vi "VI-Create XControl Event Generation.vi"(0 "Path":path=path "C:/Users/hancock/Desktop/Test/Test.xctl", 11 "error in (no error)":errorcluster) -> (15 "error out":errorcluster)   [LabVIEW 2015]
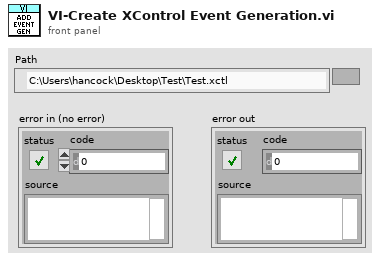
[diagram p1: front panel]
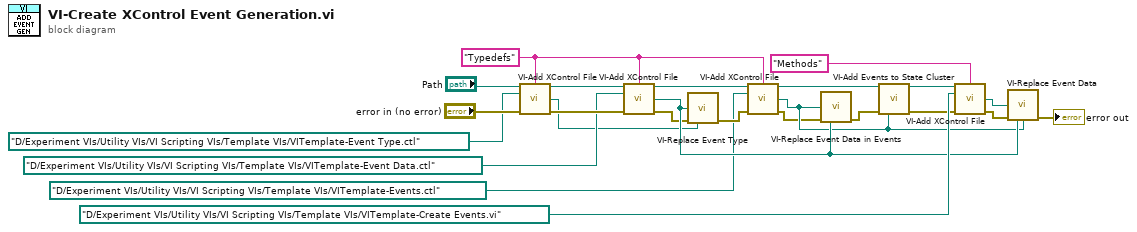
[diagram p0: block diagram]
diagram:
  w4 = "Typedefs"
  n1 = call "VI-Add XControl File.vi"("XCtl Path in"="Path", "Add to folder"=w4, "Template"=path "D:/Experiment VIs/Utility VIs/VI Scripting VIs/Template VIs/VITemplate-Event Type.ctl", "error in (no error)"="error in (no error)") -> ("XCtl Path out"=w12:path, "local path"=w8:path, "error out"=w11:errorcluster)  [unwired: 9 in]
  n2 = call "VI-Add XControl File.vi"("XCtl Path in"=w12, "Add to folder"=w4, "Template"=path "D:/Experiment VIs/Utility VIs/VI Scripting VIs/Template VIs/VITemplate-Event Data.ctl", "error in (no error)"=w11) -> ("XCtl Path out"=w7:path, "local path"=w17:path, "error out"=w9:errorcluster)  [unwired: 9 in]
  n3 = call "VI-Replace Event Type.vi"("Event Data typedef"=w17, "error in (no error)"=w9, "Event Type typedef"=w8) -> ("error out"=w6:errorcluster)  [unwired: 12 in]
  n4 = call "VI-Add XControl File.vi"("XCtl Path in"=w7, "Add to folder"=w4, "Template"=path "D:/Experiment VIs/Utility VIs/VI Scripting VIs/Template VIs/VITemplate-Events.ctl", "error in (no error)"=w6) -> ("XCtl Path out"=w1:path, "local path"=w16:path, "error out"=w3:errorcluster)  [unwired: 9 in]
  n5 = call "VI-Replace Event Data in Events.vi"("Events typedef"=w16, "error in (no error)"=w3, "Event Data typedef"=w17) -> ("error out"=w2:errorcluster)  [unwired: 12 in]
  n6 = call "VI-Add Events to State Cluster.vi"("XCtl Path in"=w1, "error in (no error)"=w2, "Event Data typedef"=w16) -> ("XCtl Path out"=w19:path, "error out"=w18:errorcluster)  [unwired: 11 in]
  n7 = call "VI-Add XControl File.vi"("XCtl Path in"=w19, "Add to folder"="Methods", "Template"=path "D:/Experiment VIs/Utility VIs/VI Scripting VIs/Template VIs/VITemplate-Create Events.vi", "error in (no error)"=w18) -> ("local path"=w22:path, "error out"=w21:errorcluster)  [unwired: 9 in, 1 out]
  n8 = call "VI-Replace Event Data.vi"("Create Events method"=w22, "error in (no error)"=w21, "Event Data typedef"=w17, "Events typedef"=w16) -> ("error out"=→"error out":errorcluster)  [unwired: 11 in]
